vi "read_ss_with_header.vi"(11 "Transpose Data Array":bool, 13 "file (use dialog)":path) -> (4 "Header String":string, 8 "Data Read":dbl[][](array[numeric]) format="%.2f", 15 "cancelled":bool)   [LabVIEW 2016]
doc: "Opens a file from the path input and reads a text header and a 2D array.\n\nThe parser string is [CR, CR, DDD, CR, CR].\n\nMuhannad Alghamdi\nPhysics 350"
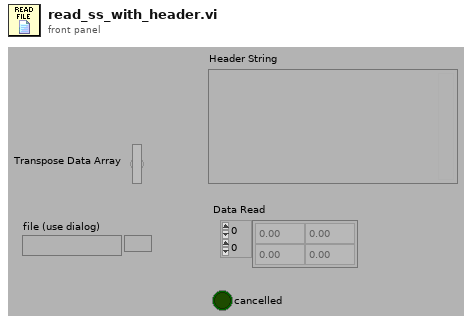
[diagram p1: front panel]
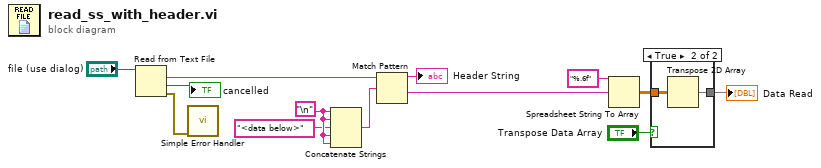
[diagram p0: block diagram]
diagram:
  w6 = "\n"
  n1 = Read from Text File(file (use dialog)="file (use dialog)") -> (text=w4:string, cancelled=→"cancelled":bool, error out=w2:errorcluster)  [unwired: 3 in, 1 out]
  n2 = call <vilib>:"Simple Error Handler.vi"("error in (no error)"=w2) -> ()  [unwired: 4 in, 5 out]
  n3 = Concatenate Strings(w6, w6, "<data below>", w6, w6) -> (w13:string)
  n4 = Match Pattern(string=w4, regular expression=w13) -> (before substring=→"Header String":string, after substring=w11:string)  [unwired: 1 in, 2 out]
  n5 = Spreadsheet String To Array(format string="%.6f", spreadsheet string=w11) -> (array=w9:dbl[][])  [unwired: 2 in]
  n6 = case shown="True" "Transpose Data Array" {
    tunnel: w9 -> [w14 w16]
    tunnel: [w14 w15] -> w7
    frame False {
    }
    frame True {
      n7 = Transpose 2D Array(2D array=w16) -> (transposed array=w15:dbl[][])
    }
  }
  "Data Read" <- w7
